vi "Launch Root Model.vi"(8 "error in (no error)":errorcluster, 11 "IViewModel In":refnum<class "IViewModel.lvclass">) -> (0 "error out":errorcluster, 3 "IViewModel Out":refnum<class "IViewModel.lvclass">)   [LabVIEW 2020, in "IViewModel.lvlib" / "IViewModel.lvclass"]
doc: "启动根模型"
uses:
  IViewModel.lvclass
  C:/Program Files/National Instruments/LabVIEW 2020/vi.lib/ActorFramework/Actor/Actor.lvclass
  IViewModel.lvclass/IViewModel.ctl
  mva-core/Source/IModel/IModel/IModel.lvclass/IModel.ctl
  mva-core/Source/IObserver/IObserver/IObserver.lvclass/IObserver.ctl
  mva-core/Source/IMediator/IMediator/IMediator.lvclass
  mva-core/Source/IModel/IModel/IModel.lvclass
  <vilib>/ActorFramework/Actor/Actor.lvclass
  mva-core/Source/IObserver/IObserver/IObserver.lvclass
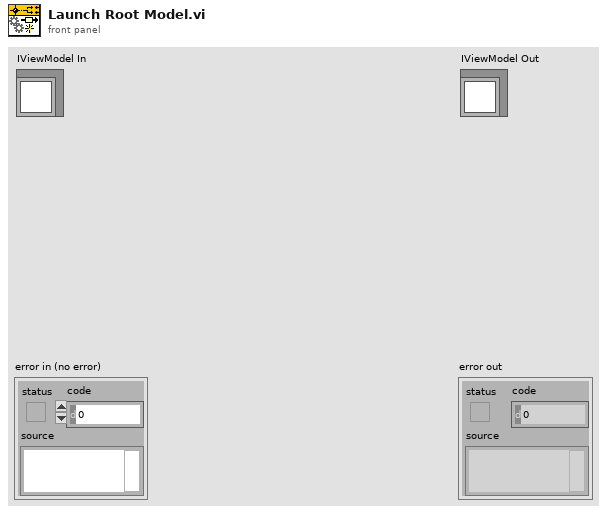
[diagram p1: front panel]
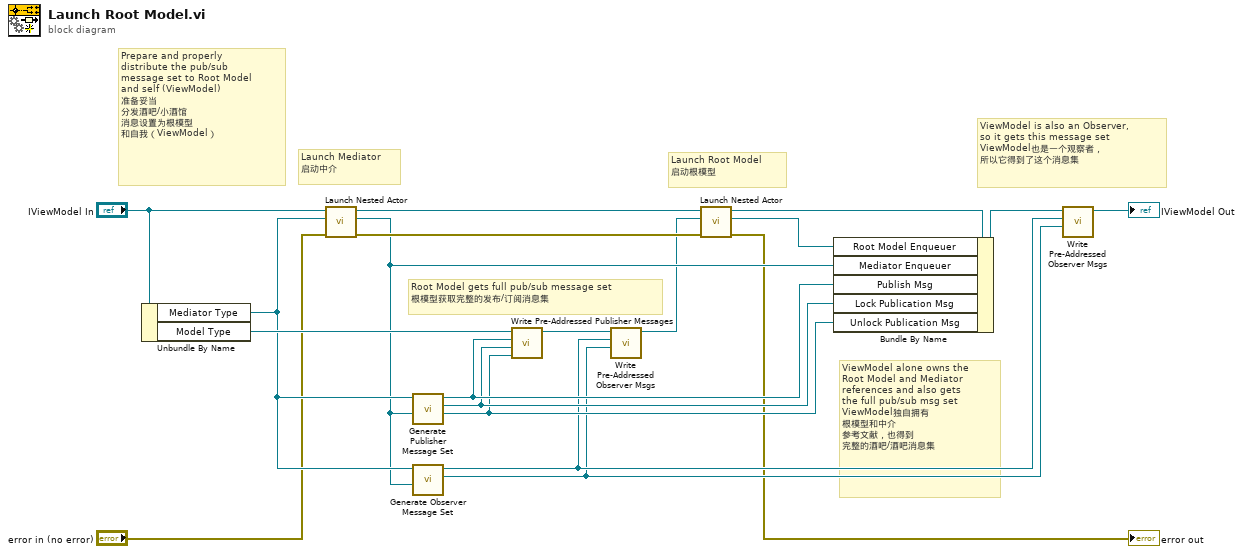
[diagram p0: block diagram]
diagram:
  # "ViewModel is also an Observer,\nso it gets this message set\nViewModel也是一个观察者，\n所以它得到了这个消息集"
  # "Root Model gets full pub/sub message set\n根模型获取完整的发布/订阅消息集"
  # "Prepare and properly\ndistribute the pub/sub\nmessage set to Root Model\nand self (ViewModel)\n准备妥当\n分发酒吧/小酒馆\n消息设置为根模型\n和自我（ViewModel）"
  # "Launch Root Model\n启动根模型"
  # "Launch Mediator\n启动中介"
  # "ViewModel alone owns the\nRoot Model and Mediator\nreferences and also gets\nthe full pub/sub msg set\nViewModel独自拥有\n根模型和中介\n参考文献，也得到\n完整的酒吧/酒吧消息集"
  n1 = Unbundle By Name("IViewModel In") -> ("Mediator Type"=w10:refnum<class "IMediator.lvclass">, "Model Type"=w17:refnum<class "IModel.lvclass">)
  n2 = call <vilib>:"Launch Nested Actor.vi"("error in (no error)"="error in (no error)", "Nested Actor"=w10, "Caller Actor in"="IViewModel In") -> ("error out"=w13:errorcluster, "Nested Actor's Enqueuer"=w9:refnum<class "Message Enqueuer.lvclass">, "Caller Actor out"=w18:refnum<class "IViewModel.lvclass">)  [unwired: 6 in]
  n3 = call-dynamic "Generate Publisher Message Set.vi"("Mediator Enqueuer"=w9, "IMediator in"=w10) -> ("Unlock Publication Msg"=w6:refnum<class "Unlock Publication Msg.lvclass">, "Lock Publication Msg"=w7:refnum<class "Lock Publication Msg.lvclass">, "Publish Msg"=w8:refnum<class "Publish Msg.lvclass">)  [unwired: 7 in]
  n4 = call-dynamic "Generate Observer Message Set.vi"("Mediator Enqueuer"=w9, "Mediator Type"=w10) -> ("Unsubscribe Msg"=w4:refnum<class "Unsubscribe Msg.lvclass">, "Subscribe Msg"=w5:refnum<class "Subscribe Msg.lvclass">)  [unwired: 8 in]
  n5 = call "Write Pre-Addressed Publisher Messages.vi"("Pre-Addressed Unlock Publication Msg"=w6, "Pre-Addressed Lock Publication Msg"=w7, "Pre-Addressed Publish Msg"=w8, "IModel in"=w17) -> ("IModel out"=w12:refnum<class "IModel.lvclass">)  [unwired: 7 in]
  n6 = call "Write Pre-Addressed Observer Msgs.vi"("Pre-Addressed Unsubscribe Msg"=w4, "Pre-Addressed Subscribe Msg"=w5, "IObserver In"=w12) -> ("IObserver Out"=w1:refnum<class "IModel.lvclass">)  [unwired: 8 in]
  n7 = call <vilib>:"Launch Nested Actor.vi"("error in (no error)"=w13, "Nested Actor"=w1, "Caller Actor in"=w18) -> ("error out"=→"error out":errorcluster, "Nested Actor's Enqueuer"=w14:refnum<class "Message Enqueuer.lvclass">, "Caller Actor out"=w16:refnum<class "IViewModel.lvclass">)  [unwired: 6 in]
  n8 = Bundle By Name(cluster=w16, "Root Model Enqueuer"=w14, "Mediator Enqueuer"=w9, "Publish Msg"=w8, "Lock Publication Msg"=w7, "Unlock Publication Msg"=w6) -> (w15:refnum<class "IViewModel.lvclass">)
  n9 = call "Write Pre-Addressed Observer Msgs.vi"("Pre-Addressed Unsubscribe Msg"=w4, "Pre-Addressed Subscribe Msg"=w5, "IObserver In"=w15) -> ("IObserver Out"=→"IViewModel Out":refnum<class "IViewModel.lvclass">)  [unwired: 8 in]
